vi "testParseStateQueueErrorTest2_2024.vi"(8 "error in (no error)":errorcluster, 11 "testStateMachineUtilities in":refnum<class "testStateMachineUtilities.lvclass">) -> (0 "error out":errorcluster, 3 "testStateMachineUtilities out":refnum<class "testStateMachineUtilities.lvclass">)   [LabVIEW 2020, in "testStateMachineUtilities.lvclass"]
uses:
  testStateMachineUtilities.lvclass
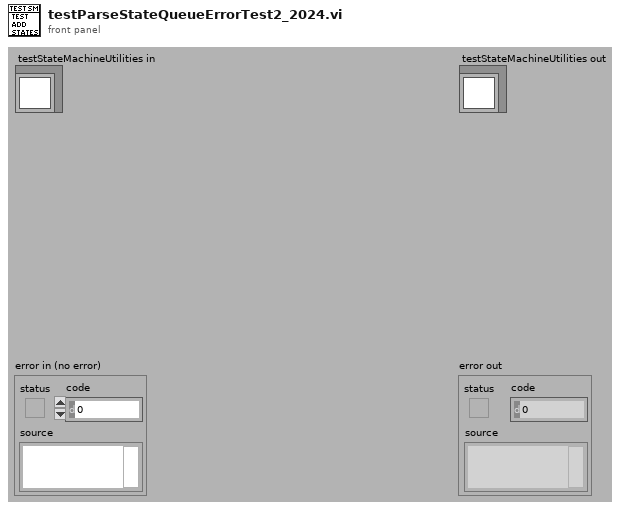
[diagram p1: front panel]
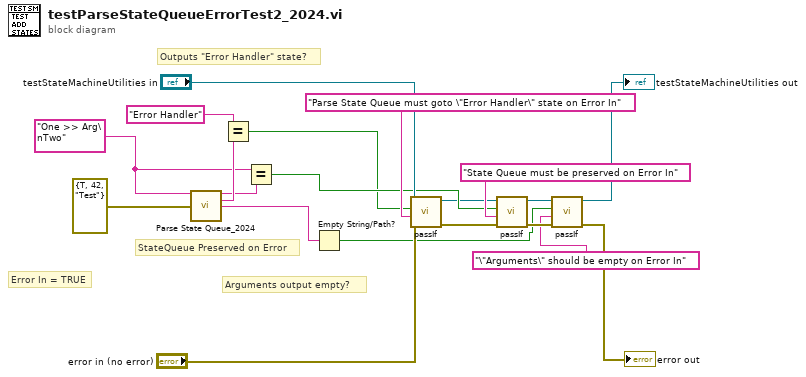
[diagram p0: block diagram]
diagram:
  w13 = "One >> Arg\nTwo" ("State Queue")
  # "Outputs \"Error Handler\" state?"
  # "Error In = TRUE"
  # "Arguments output empty?"
  # "StateQueue Preserved on Error"
  n1 = call "Parse State Queue_2024.vi"("State Queue"=w13, "Error In (no error)"=errorcluster {"status"=TRUE, "code"=42, "source"="Test"}) -> ("Remaining States"=w12:string, "Current State"=w18:string, "Arguments"=w17:string)  [unwired: 11 in]
  n2 = Equal?(x="Error Handler", y=w18) -> (x = y?=w9:bool)
  n3 = Equal?(x=w13, y=w12) -> (x = y?=w10:bool)
  n4 = Empty String/Path?(string/path=w17) -> (empty?=w5:bool)
  n5 = call-dynamic "passIf.vi"("error in (no error)"="error in (no error)", "message (\"\")"="Parse State Queue must goto \"Error Handler\" state on Error In", "pass"=w9, "TestCase in"="testStateMachineUtilities in") -> ("error out"=w2:errorcluster, "TestCase out"=w4:refnum<class "testStateMachineUtilities.lvclass">)  [unwired: 6 in]
  n6 = call-dynamic "passIf.vi"("error in (no error)"=w2, "message (\"\")"="State Queue must be preserved on Error In", "pass"=w10, "TestCase in"=w4) -> ("error out"=w8:errorcluster, "TestCase out"=w7:refnum<class "testStateMachineUtilities.lvclass">)  [unwired: 6 in]
  n7 = call-dynamic "passIf.vi"("error in (no error)"=w8, "message (\"\")"="\"Arguments\" should be empty on Error In", "pass"=w5, "TestCase in"=w7) -> ("error out"=→"error out":errorcluster, "TestCase out"=→"testStateMachineUtilities out":refnum<class "testStateMachineUtilities.lvclass">)  [unwired: 6 in]
